vi "Save.vi"(8 "error in":errorcluster, 10 "file path":path, 11 "cRIO repo in":refnum<class "cRIORepo.lvclass">) -> (0 "error out":errorcluster, 3 "cRIO repo out":refnum<class "cRIORepo.lvclass">)   [LabVIEW 2015, in "cRIORepo.lvclass"]
doc: "Calls the Read Tree VI to have an updated version of the Repo and then saves the repo information into the XML file."
uses:
  cRIORepo.lvclass
  FileCluster.ctl
  cRIORepo.lvclass/cRIORepo.ctl
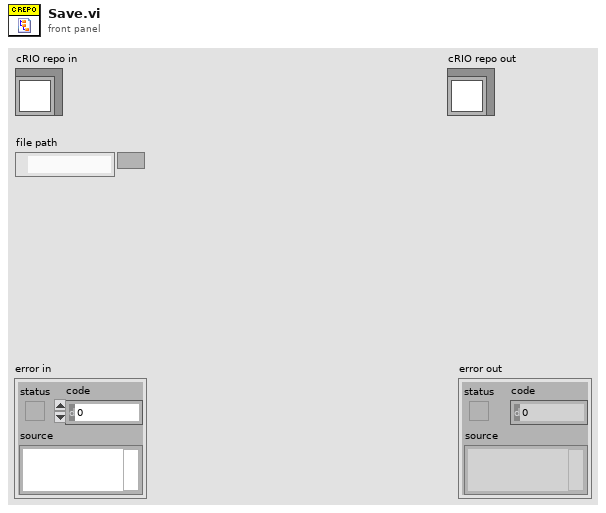
[diagram p1: front panel]
types:
  T1 = typedef "cRIORepo.lvclass/FileCluster.ctl" = cluster{"Version":string, "Data":variant}
  T2 = enum16{"open", "replace", "create", "open or create", "replace or create", "replace or create with confirmation"}
  T3 = typedef "cRIORepo.lvclass/ChannelData.ctl" = cluster{"channel group":string, "channel name":string, "IO ":string, "sensor ID":string, "description":string, "system":string, "channel type":string}
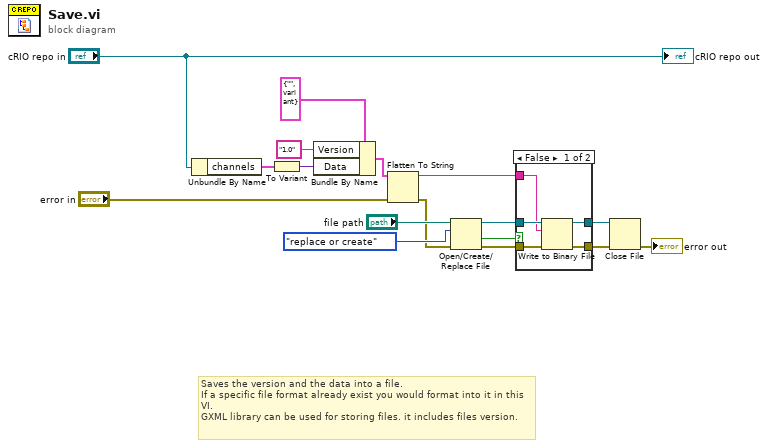
[diagram p0: block diagram]
diagram:
  # "Saves the version and the data into a file.\nIf a specific file format already exist you would format into it in this VI.\nGXML library can be used for storing files. it includes files version."
  n1 = Unbundle By Name("cRIO repo in") -> ("channels"=w15:T3[])
  n2 = To Variant(anything=w15) -> (Variant=w17:variant)
  n3 = Bundle By Name(cluster=T1 {"Version"="", "Data"=variant}, "Version"="1.0" ("Version String"), "Data"=w17) -> (w3:T1)
  n4 = Flatten To String(anything=w3, error in (no error)="error in") -> (data string=w2:string, error out=w1:errorcluster)  [unwired: 2 in, 1 out]
  n5 = Open/Create/Replace File(file path (use dialog)="file path", error in=w1, operation (0:open)=T2."replace or create") -> (refnum out=w5:refnum<file>, cancelled=w8:bool, error out=w9:errorcluster)  [unwired: 3 in]
  n6 = case shown="False" w8 {
    tunnel: w9 -> [w22 w23]
    tunnel: [w21 w23] -> w7
    tunnel: [w20 w24] -> w6
    tunnel: w5 -> [w19 w24]
    tunnel: w2 -> [w18 _]
    frame False {
      n7 = Write to Binary File(file (use dialog)=w19, data=w18, error in=w22) -> (refnum out=w20:refnum<file>, error out=w21:errorcluster)  [unwired: 3 in, 1 out]
    }
    frame True {
    }
  }
  n8 = Close File(refnum=w6, error in=w7) -> (error out=→"error out":errorcluster)  [unwired: 1 out]
  "cRIO repo out" <- "cRIO repo in"
